vi "createShutdownEvent.vi"(8 "error in (no error)":errorcluster, 11 "UserEvents in":refnum<class "UserEvents.lvclass">) -> (0 "error out":errorcluster, 3 "UserEvents out":refnum<class "UserEvents.lvclass">)   [LabVIEW 2016, in "UserEvents.lvclass"]
uses:
  UserEvents.lvclass
  Types/ShutdownEvent.ctl
  UserEvents.lvclass/UserEvents.ctl
  Types/M1M3SupportTypes.lvlib
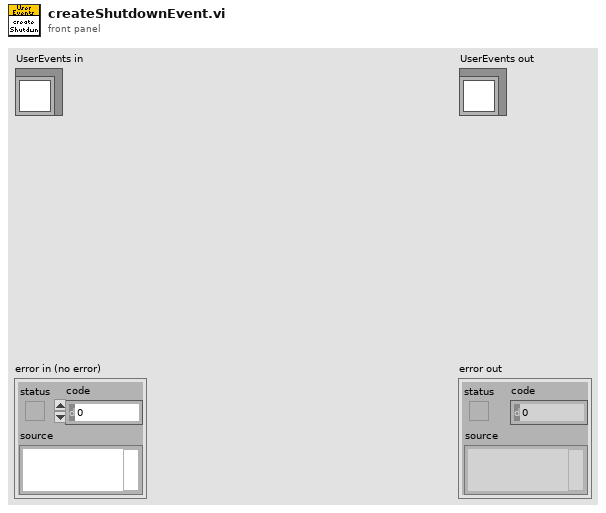
[diagram p1: front panel]
types:
  T1 = typedef "M1M3SupportTypes.lvlib/ShutdownEvent.ctl" = cluster{"Shutdown":bool}
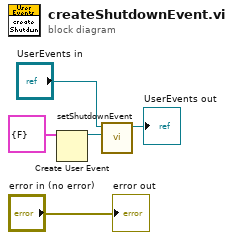
[diagram p0: block diagram]
diagram:
  n1 = Create User Event(user event datatype=T1 {"Shutdown"=FALSE} ("ShutdownEvent")) -> (user event=w4:refnum<user-event>)  [unwired: 1 in, 1 out]
  n2 = call "setShutdownEvent.vi"("ShutdownEvent"=w4, "UserEvents in"="UserEvents in") -> ("UserEvents out"=→"UserEvents out":refnum<class "UserEvents.lvclass">)  [unwired: 9 in]
  "error out" <- "error in (no error)"
